vi "Process Standard Output.vi"(8 "error in (no error)":errorcluster, 11 "Console Wrapper in":refnum<class "Console Wrapper.lvclass">) -> (0 "error out":errorcluster, 2 "Command output":string, 3 "Console Wrapper out":refnum<class "Console Wrapper.lvclass">)   [LabVIEW 2020, in "Console Wrapper.lvclass"]
doc: "Process the response for a specific command. Child classes may override this method to process what is returned. The default behavior is to display the whole command response in a dialog box."
uses:
  Console Wrapper.lvclass
  Read Standard Output.vi
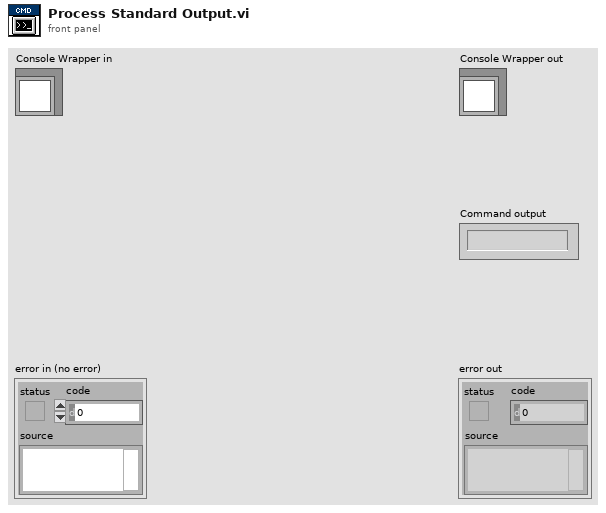
[diagram p1: front panel]
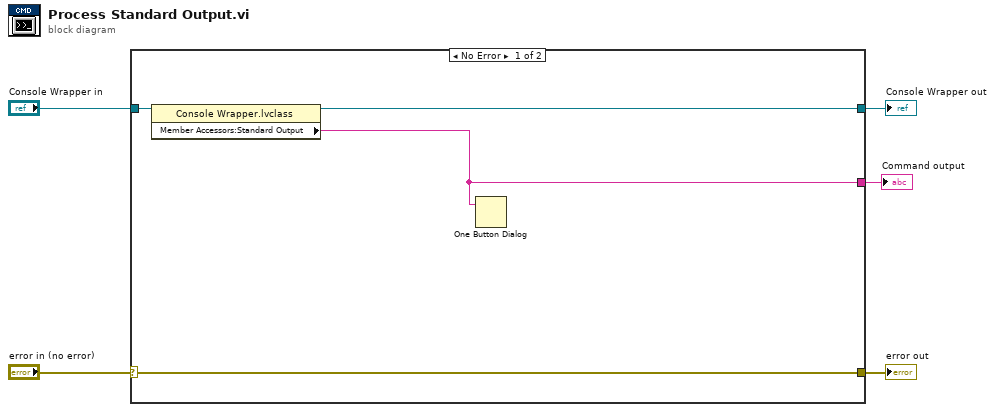
[diagram p0: block diagram]
diagram:
  n1 = case shown="No Error" "error in (no error)" {
    selector: "error in (no error)" -> [w8 w11]
    tunnel: [w8 w11] -> w4
    tunnel: [w7 w10] -> w2
    tunnel: "Console Wrapper in" -> [w9 w10]
    tunnel: [w6 _] -> w1
    frame No Error {
      n2 = property class="Console Wrapper.lvclass"(reference=w9) -> (reference out=w7:refnum<class "Console Wrapper.lvclass">, "Member Accessors:Standard Output"=w6:string)  [unwired: 1 in, 1 out]
      n3 = One Button Dialog(message=w6) -> ()  [unwired: 1 in, 1 out]
    }
    frame Error {
    }
  }
  "error out" <- w4
  "Console Wrapper out" <- w2
  "Command output" <- w1
